vi "Get DefinedName.vi"(7 "Sheet Name":string, 8 "error in":errorcluster, 10 "Range Identifier":string, 11 "SpreadsheetDoc in":refnum<k24>) -> (0 "error out":errorcluster, 2 "DefinedName":refnum<k24>, 3 "SpreadsheetDoc out":refnum<k24>, 5 "Sheet Name":string)   [LabVIEW 2019, in "Open Xml.lvlib"]
uses:
  Open Xml.lvlib
  D:/git/Open-Xml-LabVIEW/Source/DocumentFormat.OpenXml.dll
  DocumentFormat.OpenXml.dll
  D:/git/Open-Xml-LabVIEW/Source/DocumentFormat.OpenXml.Framework.dll
  DocumentFormat.OpenXml.Framework.dll
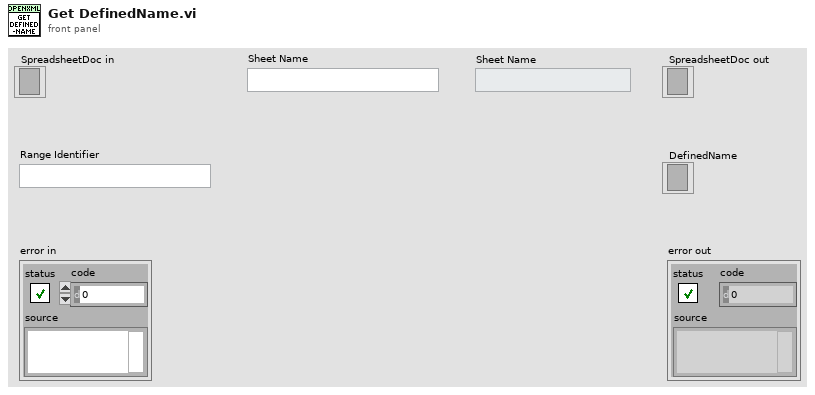
[diagram p1: front panel]
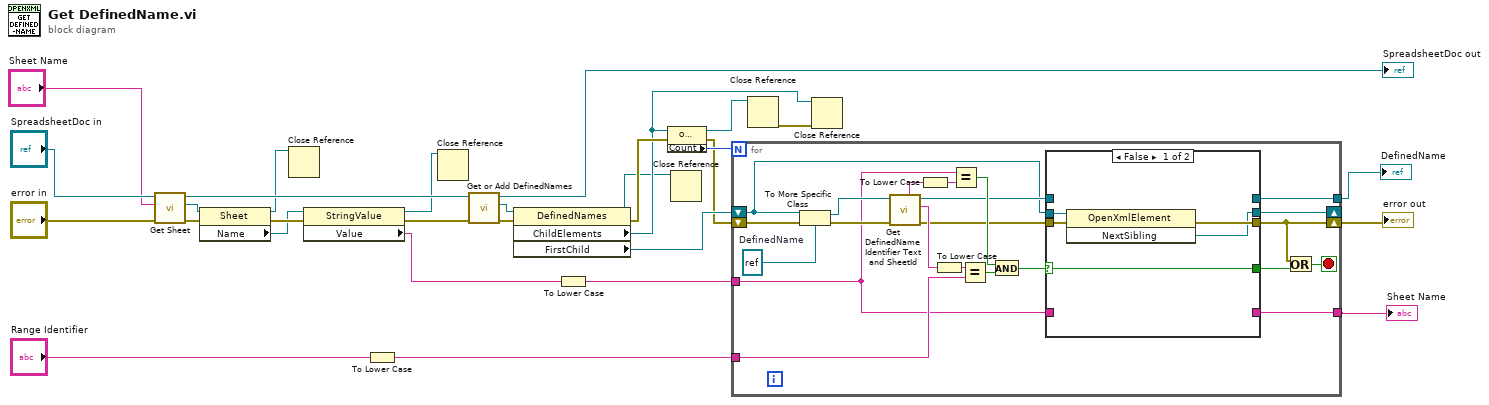
[diagram p0: block diagram]
diagram:
  n1 = call "Get Sheet.vi"("error in"="error in", "SheetName"="Sheet Name", "SpreadsheetDoc in"="SpreadsheetDoc in") -> ("error out"=w18:errorcluster, "Sheet"=w13:refnum<k24>, "SpreadsheetDoc out"=w16:refnum<k24>)  [unwired: 4 in, 2 out]
  n2 = property class="Sheet"(reference=w13, error in=w18) -> (reference out=w10:refnum<k24>, error out=w14:errorcluster, "Name"=w11:refnum<k24>)
  n3 = Close Reference(reference=w10) -> ()  [unwired: 1 in, 1 out]
  n4 = property class="StringValue"(reference=w11, error in=w14) -> (reference out=w9:refnum<k24>, error out=w12:errorcluster, "Value"=w4:string)
  n5 = To Lower Case(string="Range Identifier") -> (all lower case string=w1:string)
  n6 = Close Reference(reference=w9) -> ()  [unwired: 1 in, 1 out]
  n7 = call "Get or Add DefinedNames.vi"("error in"=w12, "SpreadsheetDoc in"=w16) -> ("error out"=w28:errorcluster, "DefinedNames"=w27:refnum<k24>, "SpreadsheetDoc out"=→"SpreadsheetDoc out":refnum<k24>)  [unwired: 7 in]
  n8 = property class="DefinedNames"(reference=w27, error in=w28) -> (reference out=w7:refnum<k24>, error out=w25:errorcluster, "ChildElements"=w21:refnum<k24>, "FirstChild"=w24:refnum<k24>)
  n9 = To Lower Case(string=w4) -> (all lower case string=w2:string)
  n10 = property class="OpenXmlElementList"(reference=w21, error in=w25) -> (reference out=w23:refnum<k24>, error out=w22:errorcluster, "Count"=w26:i32)
  n11 = Close Reference(reference=w7) -> ()  [unwired: 1 in, 1 out]
  n12 = for {
    N: w26 -> [_]
    tunnel: w1 -> [w47]
    tunnel: w2 -> [w34]
    shift-right: [w42] -> w8
    shift-left: w22 -> [w51]
    shift-right: [w37] -> _
    shift-left: w24 -> [w38]
    tunnel: [w35] -> w6
    tunnel: [w33] -> w3
    stop <- w44 stop-if-true
    w36 = refnum<k24> refnum  # DefinedName
    n13 = To More Specific Class(target class=w36, reference=w38, error in=w51) -> (specific class reference=w39:refnum<k24>, error out=w50:errorcluster)
    n14 = call "Get DefinedName Identifier Text and SheetId.vi"("error in"=w50, "DefinedName in"=w39) -> ("error out"=w43:errorcluster, "Identifier"=w48:string, "DefinedName out"=w41:refnum<k24>, "Sheet Name"=w49:string)  [unwired: 5 in, 1 out]
    n15 = To Lower Case(string=w49) -> (all lower case string=w31:string)
    n16 = To Lower Case(string=w48) -> (all lower case string=w30:string)
    n17 = Equal?(x=w34, y=w31) -> (x = y?=w45:bool)
    n18 = Equal?(x=w30, y=w47) -> (x = y?=w46:bool)
    n19 = And(x=w45, y=w46) -> (x .and. y?=w40:bool)
    n20 = case shown="False" w40 {
      selector: w40 -> [w52 w57]
      tunnel: w43 -> [w56 w60]
      tunnel: [w55 w60] -> w42
      tunnel: w41 -> [_ w61]
      tunnel: [w54 w59] -> w37
      tunnel: w38 -> [w53 w59]
      tunnel: [_ w61] -> w35
      tunnel: w34 -> [_ w58]
      tunnel: [_ w58] -> w33
      tunnel: [w52 w57] -> w32
      frame False {
        n21 = invoke class="OpenXmlElement" method="NextSibling"(reference=w53, error in=w56) -> (error out=w55:errorcluster, "NextSibling"=w54:refnum<k24>)  [unwired: 1 in, 1 out]
      }
      frame True {
      }
    }
    n22 = Or(x=w42, y=w32) -> (x .or. y?=w44:bool)
  }
  "error out" <- w8
  "DefinedName" <- w6
  "Sheet Name" <- w3
  n23 = Close Reference(reference=w23) -> (error out=w20:errorcluster)  [unwired: 1 in]
  n24 = Close Reference(reference=w21, error in (no error)=w20) -> ()  [unwired: 1 out]
